vi "20-15-5-2.vi"() -> ()   [LabVIEW 2025]
uses:
  <vilib>/Platform/TimedLoop/XDataNode/timing_clust.ctl
  <vilib>/Platform/TimedLoop/XDataNode/nitl_modes.ctl
  <vilib>/Platform/TimedLoop/XDataNode/wakeup.ctl
  <vilib>/rvi/Emulation/niFpgaSctlEmulationGetInTimedLoop.vi
  <vilib>/rvi/Emulation/niFpgaEmulationReportErrorSimple.vi
  <vilib>/rvi/Emulation/niFpgaGetClockAttributes.vi
  <vilib>/rvi/Emulation/niFpgaCriticalErrorInLSC.vi
  <vilib>/rvi/linearAlgebra/MatrixMultiply/simVIs/SubVI/nifxpla_MatrixMultiply_SimMatrixSizes.vi
  <vilib>/rvi/linearAlgebra/MatrixMultiply/simVIs/SubVI/nifxpla_MatrixMultiply_Sim4WireAdapterVector.vi
  <vilib>/rvi/linearAlgebra/MatrixMultiply/simVIs/SubVI/nifxpla_MatrixMultiply_SimFrameHandShake.vi
  <vilib>/rvi/linearAlgebra/MatrixMultiply/simVIs/SubVI/nifxpla_MatrixMultiply_SimEndlessCounter.vi
  <vilib>/rvi/linearAlgebra/MatrixMultiply/simVIs/SubVI/nifxpla_MatrixMultiply_SimVectorDataBuffer.vi
  <vilib>/rvi/ClientSDK/Core/DevComputerLib/Private/Multiply(dfxp64).vi
  <vilib>/rvi/ClientSDK/Core/DevComputerLib/Private/Dfxp128ToDfxp256.vi
  <vilib>/rvi/ClientSDK/Core/DevComputerLib/Private/Add(dfxp256).vi
  <vilib>/rvi/ClientSDK/Core/DevComputerLib/Private/Subtract(dfxp256).vi
  <vilib>/rvi/ClientSDK/Core/DevComputerLib/Private/ToDfxp64(dfxp256).vi
  <vilib>/platform/TimedLoop/XDataNode/XDataNode.xnode
  <vilib>/rvi/linearAlgebra/MatrixMultiply/XNode/nifxpla_MatrixMultiply.xnode
  <vilib>/rvi/linearAlgebra/MatrixMultiply/simVIs/nifxpla_MatrixMultiply_SimTemplateEinEout.vi
  <vilib>/rvi/linearAlgebra/MatrixMultiply/simVIs/nifxpla_MatrixMultiply_SimTemplateEinVout.vi
  <vilib>/rvi/linearAlgebra/MatrixMultiply/simVIs/nifxpla_MatrixMultiply_SimTemplateVinEout.vi
  <vilib>/rvi/linearAlgebra/MatrixMultiply/simVIs/nifxpla_MatrixMultiply_SimTemplateVinVout.vi
  <vilib>/Platform/TimedLoop/XDataNode/XDNodeRunTimeDep.lvlib
panel:
  out "Latency":u32
  out "Cycle Count 3":i32
  out "C3":fxp<+/-,32,16>[](array[numeric])
  out "C3+B":fxp<+/-,33,17>[](array[numeric])
  out "Cycle Count 2":i32
  out "C2":fxp<+/-,32,16>[](array[numeric])
  out "C2+B":fxp<+/-,33,17>[](array[numeric])
  out "Cycle Count":i32
  out "C1":fxp<+/-,32,16>[](array[numeric])
  out "C1+B":fxp<+/-,33,17>[](array[numeric])
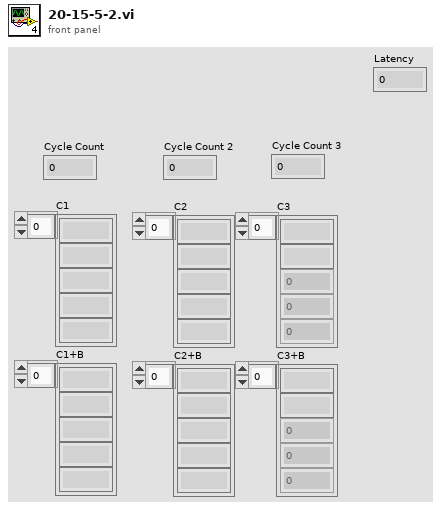
[diagram p1: front panel]
types:
  T1 = typedef "XDNodeRunTimeDep.lvlib/timing_clust.ctl" = cluster{"Expected End [f-1]":u64, "Actual End [f-1]":u64, "Finished Late? [f-1]":bool, "Expected End [i-1]":u64, "Actual End [i-1]":u64, "Finished Late? [i-1]":bool, "Expected Start [i]":u64, "Actual Start [i]":u64, "Expected Start [f]":u64, "Actual Start [f]":u64, "Source Name":string, "Structure Name":string, "Period":i64, "Deadline":i64, "Offset":i64, "Start":i64, "Priority":i32, "Timeout":i32, "Mode":T2, "Wakeup Reason":T3, "Error":errorcluster, "Source Type":string, "Secondary Source Type":string, "Global End Time":u64, "Global Start Time":u64, "Frame Duration":u64, "Iteration Duration":u64, "Assigned CPU":i32, "I/O Scan Engine Mode":u32}
  T2 = typedef "XDNodeRunTimeDep.lvlib/nitl_modes.ctl" = enum32{"No Change", "Process missed periods, maintain original phase", "Discard missed periods, maintain original phase", "Process missed periods, ignore original phase", "Discard missed periods, ignore original phase"}
  T3 = typedef "XDNodeRunTimeDep.lvlib/wakeup.ctl" = enum32{"Normal", "Aborted", "Asynchronous wakeup", "Timing source error", "Timed loop error", "Timeout"}
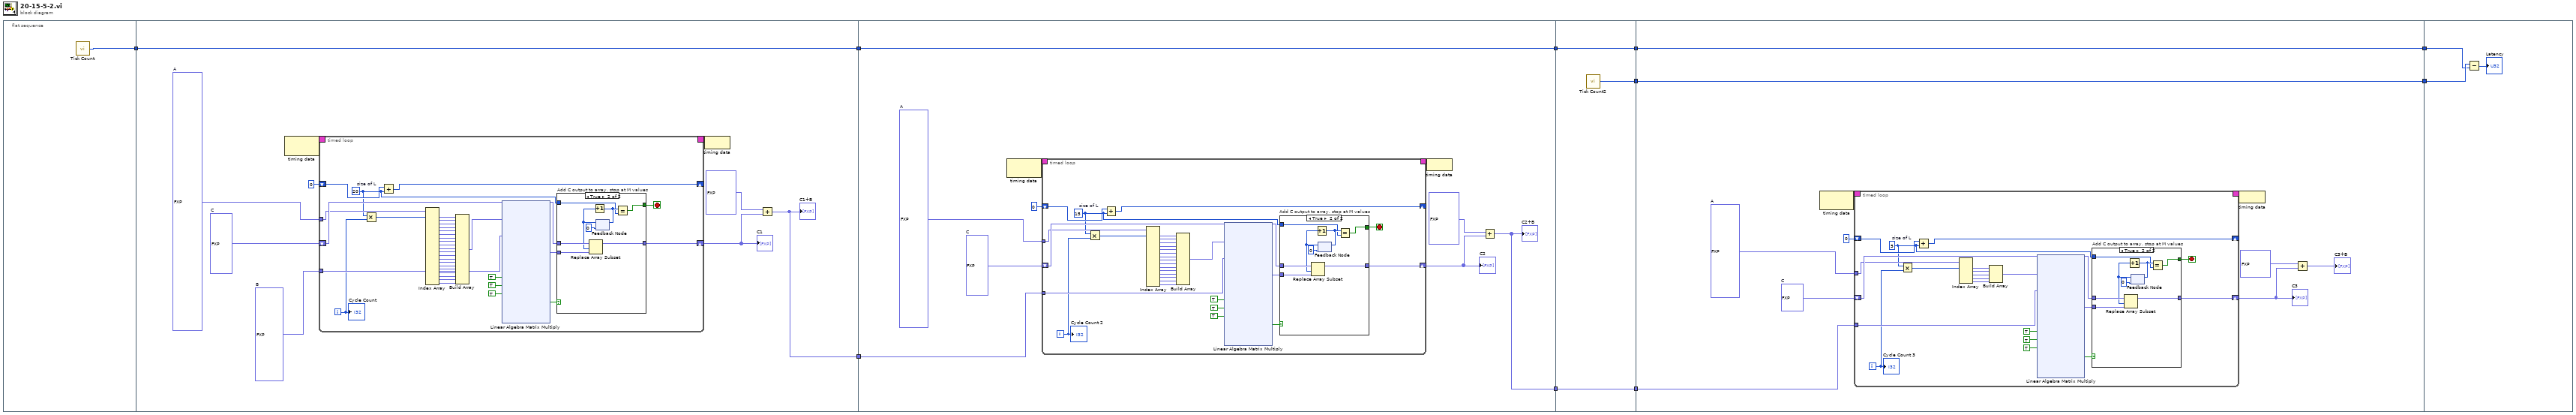
[diagram p0: block diagram]
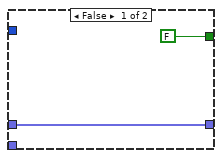
[diagram p2: hidden frame]
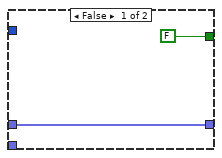
[diagram p3: hidden frame]
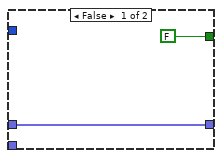
[diagram p4: hidden frame]
diagram:
  n1 = flat-sequence {
    tunnel: [w11] -> w10
    tunnel: [w13] -> w9
    tunnel: [w12] -> w8
    tunnel: w10 -> [w12]
    tunnel: w9 -> [w74]
    tunnel: [w73] -> w7
    tunnel: w8 -> [w72]
    tunnel: [w72] -> w6
    tunnel: w7 -> [w129]
    tunnel: [w129] -> w5
    tunnel: w6 -> [w128]
    tunnel: [w128] -> w4
    tunnel: [w127] -> w3
    tunnel: w5 -> [w132]
    tunnel: w4 -> [w131]
    tunnel: [w131] -> w2
    tunnel: [w130] -> w1
    tunnel: w3 -> [w130]
    tunnel: w2 -> [w177]
    tunnel: w1 -> [w178]
    frame #0 {
      n2 = call "Tick Count"() -> ("Tick Count(Ticks)"=w11:u32)
    }
    frame #1 {
      w17 = fxp<+/-,32,16>[] [0.0, 0.0, 0.0, 0.0, 0.0, 0.0, 0.0, 0.0, 0.0, 0.0, 0.0, 0.0, 0.0, 0.0, 0.0, 0.0, 0.0, 0.0, 0.0, 0.0, 0.0, 0.0, 0.0, 0.0, 0.0, 0.0, 0.0, 0.0, 0.0, 0.0, 0.0, 0.0, 0.0, 0.0, 0.0, 0.0, 0.0, 0.0, 0.0, 0.0, 0.0, 0.0, 0.0, 0.0, 0.0, 0.0, 0.0, 0.0, 0.0, 0.0, 0.0, 0.0, 0.0, 0.0, 0.0, 0.0, 0.0, 0.0, 0.0, 0.0, 0.0, 0.0, 0.0, 0.0, 0.0, 0.0, 0.0, 0.0, 0.0, 0.0, 0.0, 0.0, 0.0, 0.0, 0.0, 0.0, 0.0, 0.0, 0.0, 0.0, 0.0, 0.0, 0.0, 0.0, 0.0, 0.0, 0.0, 0.0, 0.0, 0.0, 0.0, 0.0, 0.0, 0.0, 0.0, 0.0, 0.0, 0.0, 0.0, 0.0, 0.0, 0.0, 0.0, 0.0, 0.0, 0.0, 0.0, 0.0, 0.0, 0.0, 0.0, 0.0, 0.0, 0.0, 0.0, 0.0, 0.0, 0.0, 0.0, 0.0, 0.0, 0.0, 0.0, 0.0, 0.0, 0.0, 0.0, 0.0, 0.0, 0.0, 0.0, 0.0, 0.0, 0.0, 0.0, 0.0, 0.0, 0.0, 0.0, 0.0, 0.0, 0.0, 0.0, 0.0, 0.0, 0.0, 0.0, 0.0, 0.0, 0.0, 0.0, 0.0, 0.0, 0.0, 0.0, 0.0, 0.0, 0.0, 0.0, 0.0, 0.0, 0.0, 0.0, 0.0, 0.0, 0.0, 0.0, 0.0, 0.0, 0.0, 0.0, 0.0, 0.0, 0.0, 0.0, 0.0, 0.0, 0.0, 0.0, 0.0, 0.0, 0.0, 0.0, 0.0, 0.0, 0.0, 0.0, 0.0, 0.0, 0.0, 0.0, 0.0, 0.0, 0.0, 0.0, 0.0, 0.0, 0.0, 0.0, 0.0, 0.0, 0.0, 0.0, 0.0, 0.0, 0.0, 0.0, 0.0, 0.0, 0.0, 0.0, 0.0, 0.0, 0.0, 0.0, 0.0, 0.0, 0.0, 0.0, 0.0, 0.0, 0.0, 0.0, 0.0, 0.0, 0.0, 0.0, 0.0, 0.0, 0.0, 0.0, 0.0, 0.0, 0.0, 0.0, 0.0, 0.0, 0.0, 0.0, 0.0, 0.0, 0.0, 0.0, 0.0, 0.0, 0.0, 0.0, 0.0, 0.0, 0.0, 0.0, 0.0, 0.0, 0.0, 0.0, 0.0, 0.0, 0.0, 0.0, 0.0, 0.0, 0.0, 0.0, 0.0, 0.0, 0.0, 0.0, 0.0, 0.0, 0.0, 0.0, 0.0, 0.0, 0.0, 0.0, 0.0, 0.0, 0.0, 0.0, 0.0, 0.0, 0.0, 0.0, 0.0, 0.0, 0.0, 0.0, 0.0, 0.0, 0.0, 0.0, 0.0, 0.0, 0.0, 0.0, 0.0, 0.0, 0.0, 0.0, 0.0]  # A
      w18 = fxp<+/-,32,16>[] [0.0, 0.0, 0.0, 0.0, 0.0, 0.0, 0.0, 0.0, 0.0, 0.0, 0.0, 0.0, 0.0, 0.0, 0.0, 0.0, 0.0, 0.0, 0.0, 0.0]  # B
      w19 = fxp<+/-,32,16>[] [0.0, 0.0, 0.0, 0.0, 0.0, 0.0, 0.0, 0.0, 0.0, 0.0, 0.0, 0.0, 0.0, 0.0, 0.0]  # C
      n3 = node-c288() -> (w21:T1)  [unwired: 1 in]
      n4 = timed-loop {
        timing: w21 -> [_]
        timing-out: [_] -> w20
        shift-right: [w56] -> w15
        shift-left: w19 -> [w55]
        tunnel: w18 -> [w52]
        tunnel: w17 -> [w35]
        shift-right: [w48] -> _
        shift-left: 0 ("length") -> [w49]
        i -> [w34]
        stop <- w54 stop-if-true
        w33 = 20  # size of L
        n5 = Multiply(x=w33, y=w34) -> (x*y=w46:i32)
        n6 = Add(x=w49, y=w33) -> (x+y=w48:i32)
        n7 = Index Array(array=w35, index #1=w46) -> (element #1=w45:fxp<+/-,32,16>, element #2=w44:fxp<+/-,32,16>, element #3=w43:fxp<+/-,32,16>, element #4=w42:fxp<+/-,32,16>, element #5=w41:fxp<+/-,32,16>, element #6=w40:fxp<+/-,32,16>, element #7=w39:fxp<+/-,32,16>, element #8=w38:fxp<+/-,32,16>, element #9=w37:fxp<+/-,32,16>, element #10=w36:fxp<+/-,32,16>, element #11=w31:fxp<+/-,32,16>, element #12=w30:fxp<+/-,32,16>, element #13=w29:fxp<+/-,32,16>, element #14=w28:fxp<+/-,32,16>, element #15=w27:fxp<+/-,32,16>, element #16=w26:fxp<+/-,32,16>, element #17=w25:fxp<+/-,32,16>, element #18=w24:fxp<+/-,32,16>, element #19=w23:fxp<+/-,32,16>, element #20=w22:fxp<+/-,32,16>)  [unwired: 19 in]
        n8 = Build Array(w45, w44, w43, w42, w41, w40, w39, w38, w37, w36, w31, w30, w29, w28, w27, w26, w25, w24, w23, w22) -> (w32:fxp<+/-,32,16>[])
        n9 = xnode ("Linear Algebra Matrix Multiply")("ar"=w32, "br"=w52, "a valid"=TRUE, "b valid"=TRUE, "ready for output (T)"=TRUE) -> ("cr"=w51:fxp<+/-,64,37>[], "output valid"=w47:bool)  [unwired: 2 in, 4 out]
        n10 = case "Add C output to array, stop at M values" shown="True" w47 {
          tunnel: w51 -> [_ w63]
          tunnel: [w59 w66] -> w56
          tunnel: w55 -> [w59 w67]
          tunnel: [FALSE w64] -> w54
          tunnel: w33 -> [_ w60]
          frame False {
          }
          frame True {
            n11 = feedback #1(0 ("x")) -> (w62:i32)
            n12 = Replace Array Subset(array=w67, new element=w63, index=w62) -> (w66:fxp<+/-,32,16>[])
            n13 = Increment(x=w62) -> (x+1=w61:i32)
            n14 = feedback-in #1(w61) -> ()
            n15 = Equal?(x=w61, y=w60) -> (x = y?=w64:bool)
          }
        }
        "Cycle Count" <- w34
      }
      "C1" <- w15
      n16 = node-c288(w20) -> ()
      n17 = Add(x=fxp<+/-,32,16>[] [0.5, 0.5, 0.5, 0.5, 0.5, 0.0, 0.0, 0.0, 0.0, 0.0, 0.0, 0.0, 0.0, 0.0, 0.0], y=w15) -> (x+y=w13:fxp<+/-,33,17>[])
      "C1+B" <- w13
    }
    frame #2 {
      w78 = fxp<+/-,32,16>[] [0.0, 0.0, 0.0, 0.0, 0.0, 0.0, 0.0, 0.0, 0.0, 0.0, 0.0, 0.0, 0.0, 0.0, 0.0, 0.0, 0.0, 0.0, 0.0, 0.0, 0.0, 0.0, 0.0, 0.0, 0.0, 0.0, 0.0, 0.0, 0.0, 0.0, 0.0, 0.0, 0.0, 0.0, 0.0, 0.0, 0.0, 0.0, 0.0, 0.0, 0.0, 0.0, 0.0, 0.0, 0.0, 0.0, 0.0, 0.0, 0.0, 0.0, 0.0, 0.0, 0.0, 0.0, 0.0, 0.0, 0.0, 0.0, 0.0, 0.0, 0.0, 0.0, 0.0, 0.0, 0.0, 0.0, 0.0, 0.0, 0.0, 0.0, 0.0, 0.0, 0.0, 0.0, 0.0]  # A
      w79 = fxp<+/-,32,16>[] [0.0, 0.0, 0.0, 0.0, 0.0]  # C
      n18 = node-c288() -> (w81:T1)  [unwired: 1 in]
      n19 = timed-loop {
        timing: w81 -> [_]
        timing-out: [_] -> w80
        shift-right: [w111] -> w76
        shift-left: w79 -> [w110]
        tunnel: w74 -> [w107]
        tunnel: w78 -> [w95]
        shift-right: [w103] -> _
        shift-left: 0 ("length") -> [w104]
        i -> [w94]
        stop <- w109 stop-if-true
        w93 = 15  # size of L
        n20 = Multiply(x=w93, y=w94) -> (x*y=w101:i32)
        n21 = Add(x=w104, y=w93) -> (x+y=w103:i32)
        n22 = Index Array(array=w95, index #1=w101) -> (element #1=w100:fxp<+/-,32,16>, element #2=w99:fxp<+/-,32,16>, element #3=w98:fxp<+/-,32,16>, element #4=w97:fxp<+/-,32,16>, element #5=w96:fxp<+/-,32,16>, element #6=w91:fxp<+/-,32,16>, element #7=w90:fxp<+/-,32,16>, element #8=w89:fxp<+/-,32,16>, element #9=w88:fxp<+/-,32,16>, element #10=w87:fxp<+/-,32,16>, element #11=w86:fxp<+/-,32,16>, element #12=w85:fxp<+/-,32,16>, element #13=w84:fxp<+/-,32,16>, element #14=w83:fxp<+/-,32,16>, element #15=w82:fxp<+/-,32,16>)  [unwired: 14 in]
        n23 = Build Array(w100, w99, w98, w97, w96, w91, w90, w89, w88, w87, w86, w85, w84, w83, w82) -> (w92:fxp<+/-,32,16>[])
        n24 = xnode ("Linear Algebra Matrix Multiply")("ar"=w92, "br"=w107, "a valid"=TRUE, "b valid"=TRUE, "ready for output (T)"=TRUE) -> ("cr"=w106:fxp<+/-,64,37>[], "output valid"=w102:bool)  [unwired: 2 in, 4 out]
        n25 = case "Add C output to array, stop at M values" shown="True" w102 {
          tunnel: w106 -> [_ w118]
          tunnel: [w114 w121] -> w111
          tunnel: w110 -> [w114 w122]
          tunnel: [FALSE w119] -> w109
          tunnel: w93 -> [_ w115]
          frame False {
          }
          frame True {
            n26 = feedback #2(0 ("x")) -> (w117:i32)
            n27 = Replace Array Subset(array=w122, new element=w118, index=w117) -> (w121:fxp<+/-,32,16>[])
            n28 = Increment(x=w117) -> (x+1=w116:i32)
            n29 = feedback-in #2(w116) -> ()
            n30 = Equal?(x=w116, y=w115) -> (x = y?=w119:bool)
          }
        }
        "Cycle Count 2" <- w94
      }
      "C2" <- w76
      n31 = node-c288(w80) -> ()
      n32 = Add(x=fxp<+/-,32,16>[] [0.5, 0.5, 0.5, 0.5, 0.5], y=w76) -> (x+y=w73:fxp<+/-,33,17>[])
      "C2+B" <- w73
    }
    frame #3 {
      n33 = call "Tick Count2"() -> ("Tick Count(Ticks)"=w127:u32)
    }
    frame #4 {
      w137 = fxp<+/-,32,16>[] [0.0, 0.0, 0.0, 0.0, 0.0, 0.0, 0.0, 0.0, 0.0, 0.0]  # A
      w138 = fxp<+/-,32,16>[] [0.0, 0.0]  # C
      n34 = node-c288() -> (w140:T1)  [unwired: 1 in]
      n35 = timed-loop {
        timing: w140 -> [_]
        timing-out: [_] -> w139
        shift-right: [w160] -> w135
        shift-left: w138 -> [w159]
        tunnel: w132 -> [w156]
        tunnel: w137 -> [w144]
        shift-right: [w152] -> _
        shift-left: 0 ("length") -> [w153]
        i -> [w143]
        stop <- w158 stop-if-true
        w142 = 5  # size of L
        n36 = Multiply(x=w142, y=w143) -> (x*y=w150:i32)
        n37 = Add(x=w153, y=w142) -> (x+y=w152:i32)
        n38 = Index Array(array=w144, index #1=w150) -> (element #1=w149:fxp<+/-,32,16>, element #2=w148:fxp<+/-,32,16>, element #3=w147:fxp<+/-,32,16>, element #4=w146:fxp<+/-,32,16>, element #5=w145:fxp<+/-,32,16>)  [unwired: 4 in]
        n39 = Build Array(w149, w148, w147, w146, w145) -> (w141:fxp<+/-,32,16>[])
        n40 = xnode ("Linear Algebra Matrix Multiply")("ar"=w141, "br"=w156, "a valid"=TRUE, "b valid"=TRUE, "ready for output (T)"=TRUE) -> ("cr"=w155:fxp<+/-,64,36>[], "output valid"=w151:bool)  [unwired: 2 in, 4 out]
        n41 = case "Add C output to array, stop at M values" shown="True" w151 {
          tunnel: w155 -> [_ w167]
          tunnel: [w163 w170] -> w160
          tunnel: w159 -> [w163 w171]
          tunnel: [FALSE w168] -> w158
          tunnel: w142 -> [_ w164]
          frame False {
          }
          frame True {
            n42 = feedback #3(0 ("x")) -> (w166:i32)
            n43 = Replace Array Subset(array=w171, new element=w167, index=w166) -> (w170:fxp<+/-,32,16>[])
            n44 = Increment(x=w166) -> (x+1=w165:i32)
            n45 = feedback-in #3(w165) -> ()
            n46 = Equal?(x=w165, y=w164) -> (x = y?=w168:bool)
          }
        }
        "Cycle Count 3" <- w143
      }
      "C3" <- w135
      n47 = node-c288(w139) -> ()
      n48 = Add(x=fxp<+/-,32,16>[] [0.5, 0.5], y=w135) -> (x+y=→"C3+B":fxp<+/-,33,17>[])
    }
    frame #5 {
      n49 = Subtract(x=w178, y=w177) -> (x-y=→"Latency":u32)
    }
  }
